vi "Write json to Param one.vi"(8 "error in (no error)":errorcluster, 10 "JSON Data In":string, 11 "PAR in":T1) -> (0 "error out":errorcluster, 3 "PAR out":T1)   [LabVIEW 2019, in "Inputs.lvlib"]
uses:
  Inputs.lvlib
  Ctl/Param.ctl
  Ctl/ParamColumns.ctl
  <vilib>/JDP Science/JSONtext/Find Multiple Items.vi
  <vilib>/JDP Science/JSONtext/String Subset.vi
  <vilib>/JDP Science/JSONtext/support/Strip Quotes and Unescape.vi
  <vilib>/JDP Science/JSONtext/Parsing/Parse Full Path or Item Name.vi
  <vilib>/JDP Science/JSONtext/Offset/Find Item Locations by Path.vi
  <vilib>/JDP Science/JSONtext/support/Unescape JSON string.vi
  <vilib>/JDP Science/JSONtext/Get Array Elements.vi
  Userlib.lvlib
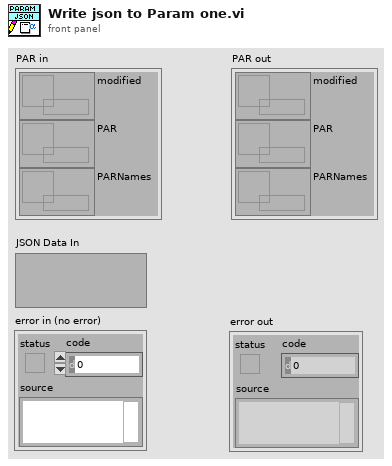
[diagram p1: front panel]
types:
  T1 = typedef "Inputs.lvlib/Param.ctl" = cluster{"modified":refnum<data-value>, "PAR":refnum<data-value>, "PARNames":refnum<data-value>}
  T2 = typedef "Inputs.lvlib/ParamColumns.ctl" = enum16{"value", "value_range_min", "value_range_max", "d", "fname", "value_units", "fcode", "fcodef", "fcode_full"}
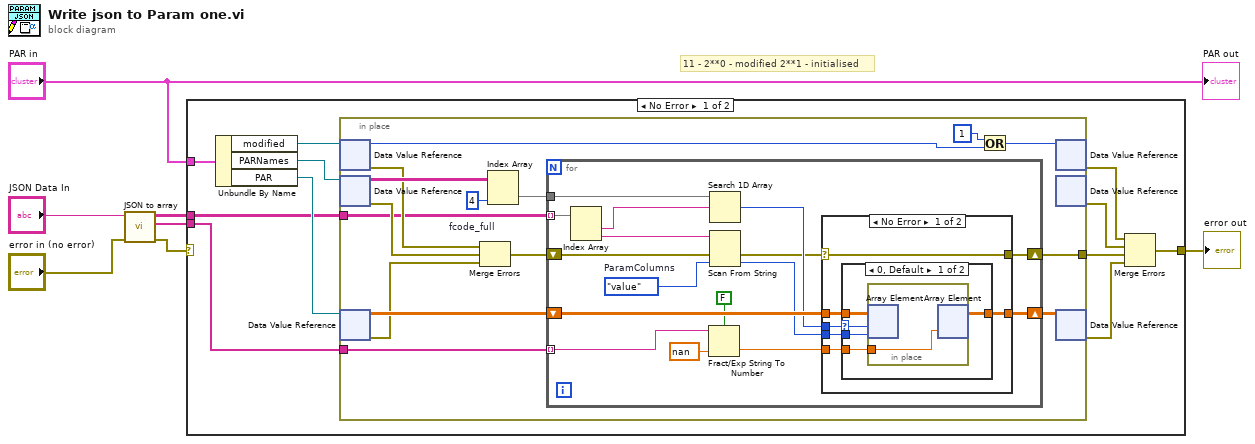
[diagram p0: block diagram]
diagram:
  # "11 - 2**0 - modified 2**1 - initialised"
  n1 = call "JSON to array.vi"("error in (no error)"="error in (no error)", "JSON Data In"="JSON Data In") -> ("error out"=w4:errorcluster, "values"=w1:string[], "names"=w2:string[][])  [unwired: 7 in]
  n2 = case shown="No Error" w4 {
    selector: w4 -> [_ w65]
    tunnel: [w17 w65] -> w7
    tunnel: "PAR in" -> [w18 _]
    tunnel: w1 -> [w15 _]
    tunnel: w2 -> [w10 _]
    frame No Error {
      n3 = Unbundle By Name(w18) -> ("modified"=w12:refnum<data-value>, "PARNames"=w14:refnum<data-value>, "PAR"=w16:refnum<data-value>)
      n4 = in-place {
        in-place-border: w15 -> [w25]
        in-place-border: [w26] -> w8
        in-place-border: w10 -> [w19]
        w30 = 4  # fcode_full
        n5 = in-place-dvr #1(w12) -> (w23:u8, w21:errorcluster)
        n6 = in-place-dvr #2(w14) -> (w31:string[][], w28:errorcluster)
        n7 = in-place-dvr #3(w16) -> (w33:dbl[][], w27:errorcluster)
        n8 = Merge Errors(w21, w28, w27) -> (w20:errorcluster)
        n9 = Index Array(array=w31, index (col)=w30) -> (element=w29:string[])  [unwired: 1 in]
        n10 = for {
          tunnel: w29 -> [w47]
          tunnel: w25 -> [w42] mode=indexing
          shift-right: [w43] -> w26
          shift-left: w20 -> [w39]
          shift-right: [w48] -> w32
          shift-left: w33 -> [w49]
          tunnel: w19 -> [w37] mode=indexing
          w46 = ParamColumns."value"  # ParamColumns
          n11 = Index Array(array=w37) -> (element #1=w36:string, element #2=w35:string)  [unwired: 2 in]
          n12 = Fract/Exp String To Number(use system decimal point (T)=FALSE, string=w42, default (0 dbl)=nan ("default (0 DBL)")) -> (number=w41:dbl)  [unwired: 1 in, 1 out]
          n13 = Search 1D Array(1D array=w47, element=w36) -> (index of element=w45:i32)  [unwired: 1 in]
          n14 = Scan From String(input string=w35, error in=w39, default 1=w46) -> (error out=w38:errorcluster, output 1=w44:T2)  [unwired: 2 in, 2 out]
          n15 = case shown="No Error" w38 {
            selector: w38 -> [w50 w63]
            tunnel: w49 -> [w55 w64]
            tunnel: [w54 w64] -> w48
            tunnel: w44 -> [w53 _]
            tunnel: w41 -> [w52 _]
            tunnel: w45 -> [w51 _]
            tunnel: [w50 w63] -> w43
            frame No Error {
              n16 = case shown="0, Default" w51 {
                selector: w51 -> [w56 _]
                tunnel: w55 -> [w60 w62]
                tunnel: [w59 w62] -> w54
                tunnel: w53 -> [w58 _]
                tunnel: w52 -> [w57 _]
                frame 0, Default {
                  n17 = in-place {
                    in-place-border: w57 -> [w61]
                    n18 = in-place-array #4(w60, w56, w58) -> ()  [unwired: 1 out]
                    n19 = in-place-array #4(w61) -> (w59:dbl[][])  [unwired: 2 out]
                  }
                }
                frame -1 {
                }
              }
            }
            frame Error {
            }
          }
        }
        n20 = Or(x=u8 1 ("data value"), y=w23) -> (x .or. y?=w22:u8)
        n21 = in-place-dvr #1(w22) -> (w11:errorcluster)  [unwired: 1 out]
        n22 = in-place-dvr #2() -> (w13:errorcluster)  [unwired: 1 in, 1 out]
        n23 = in-place-dvr #3(w32) -> (w9:errorcluster)  [unwired: 1 out]
      }
      n24 = Merge Errors(w11, w13, w8, w9) -> (w17:errorcluster)
    }
    frame Error {
    }
  }
  "error out" <- w7
  "PAR out" <- "PAR in"
